vi "FV-resample-get_min_array_value.vi"(7 "min Frequency":dbl, 10 "Frequency array":dbl[](array[numeric])) -> (1 "Position":i32)   [LabVIEW 2020, in "FV-file_viewer.lvlib"]
uses:
  FV-file_viewer.lvlib
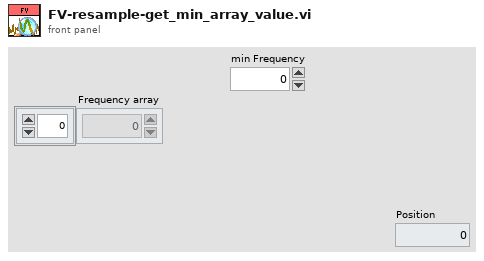
[diagram p1: front panel]
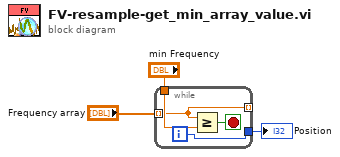
[diagram p0: block diagram]
diagram:
  n1 = while {
    tunnel: "Frequency array" -> [w5] mode=indexing
    tunnel: "min Frequency" -> [w7]
    tunnel: [w5] -> _ mode=indexing
    tunnel: [w4] -> w1
    i -> [w4]
    stop <- w6 stop-if-true
    n2 = Greater Or Equal?(x=w5, y=w7) -> (x >= y?=w6:bool)
  }
  "Position" <- w1
